vi "Get Control Information.vi"(8 "error in (no error)":errorcluster, 11 "Waveform Graph in":refnum<class "Waveform Graph.lvclass">) -> (0 "error out":errorcluster, 2 "Control Information":string[][](array[string]), 3 "Waveform Graph out":refnum<class "Waveform Graph.lvclass">)   [LabVIEW 2017, in "Localization.lvlib" / "Waveform Graph.lvclass"]
doc: "VI for override that is supposed to do go throgh the process for each control type and pull out the information that is necessary for each control.\n\nChoose Movement Consulting, LLC"
uses:
  Waveform Graph.lvclass
  C:/Apps/CMC/OpenSource/Localization/Control Info/Control Info.lvclass
  Localization.lvlib
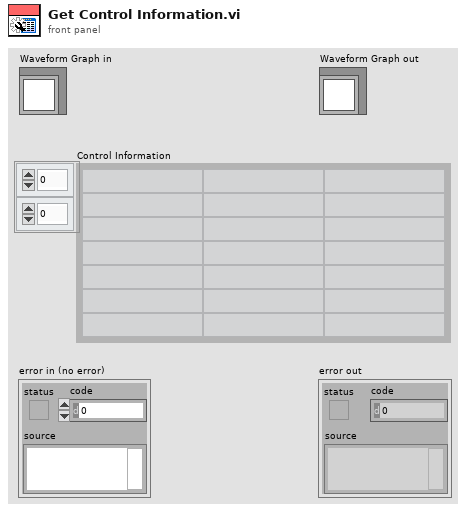
[diagram p1: front panel]
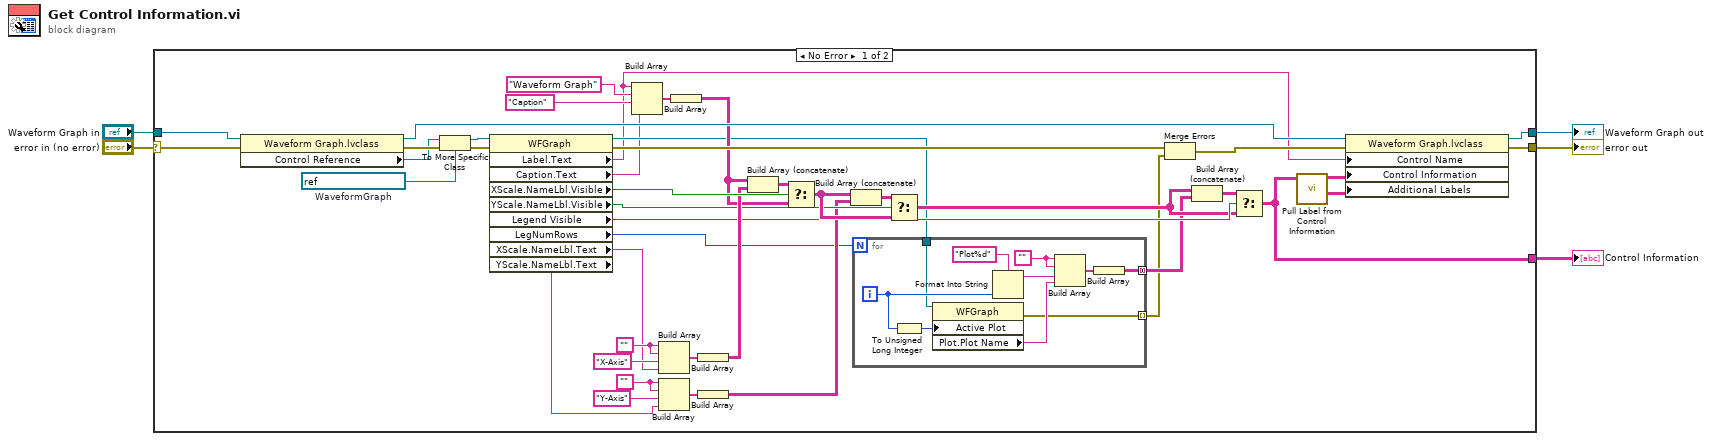
[diagram p0: block diagram]
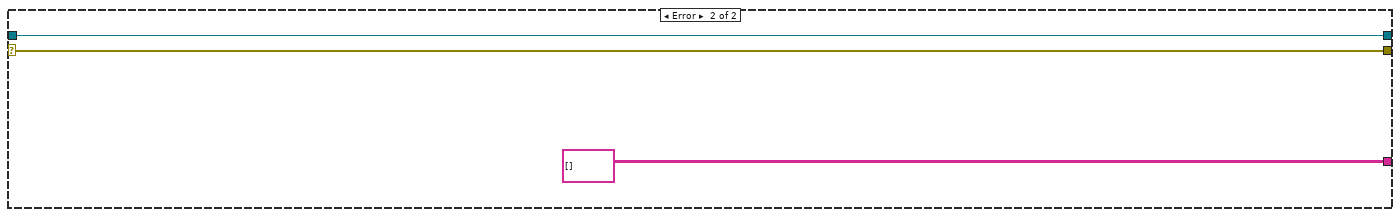
[diagram p2: hidden frame]
diagram:
  n1 = case shown="No Error" "error in (no error)" {
    selector: "error in (no error)" -> [w43 w61]
    tunnel: [w39 w61] -> w3
    tunnel: "Waveform Graph in" -> [w42 w60]
    tunnel: [w8 string[][] []] -> w2
    tunnel: [w37 w60] -> w1
    frame No Error {
      w26 = ""
      w29 = ""
      w48 = refnum<vi> refnum  # WaveformGraph
      n2 = property class="Waveform Graph.lvclass"(reference=w42, error in=w43) -> (reference out=w38:refnum<class "Waveform Graph.lvclass">, error out=w44:errorcluster, "Control Reference"=w41:refnum<vi>)
      n3 = To More Specific Class(target class=w48, reference=w41, error in=w44) -> (specific class reference=w47:refnum<vi>, error out=w45:errorcluster)
      n4 = property class="WFGraph"(reference=w47, error in=w45) -> (reference out=w13:refnum<vi>, error out=w40:errorcluster, "Label.Text"=w9:string, "Caption.Text"=w10:string, "XScale.NameLbl.Visible"=w36:bool, "YScale.NameLbl.Visible"=w22:bool, "Legend Visible"=w18:bool, "LegNumRows"=w20:u32, "XScale.NameLbl.Text"=w14:string, "YScale.NameLbl.Text"=w15:string)
      n5 = Build Array(w9, "Waveform Graph", "Caption", w10) -> (w46:string[])
      n6 = Build Array(w29, w29, "X-Axis", w14) -> (w30:string[])
      n7 = Build Array(w26, w26, "Y-Axis", w15) -> (w25:string[])
      n8 = Build Array(w46) -> (w34:string[][])
      n9 = Build Array(w30) -> (w35:string[][])
      n10 = Build Array(w25) -> (w21:string[][])
      n11 = Build Array (concatenate)(w34, w35) -> (w33:string[][])
      n12 = Select(t=w33, s=w36, f=w34) -> (s? t:f=w23:string[][])
      n13 = Build Array (concatenate)(w23, w21) -> (w24:string[][])
      n14 = for {
        N: w20 -> [_]
        tunnel: [w57] -> w16 mode=concatenating
        tunnel: w13 -> [w50]
        tunnel: [w49] -> w11 mode=indexing
        i -> [w53]
        w56 = ""
        n15 = To Unsigned Long Integer(number=w53) -> (unsigned 32bit integer=w51:u32)
        n16 = property class="WFGraph"(reference=w50, "Active Plot"=w51) -> (error out=w49:errorcluster, "Plot.Plot Name"=w52:string)  [unwired: 1 in, 1 out]
        n17 = Format Into String(format string="Plot%d", w53) -> (resulting string=w54:string)  [unwired: 2 in, 1 out]
        n18 = Build Array(w56, w56, w54, w52) -> (w58:string[])
        n19 = Build Array(w58) -> (w57:string[][])
      }
      n20 = Select(t=w24, s=w22, f=w23) -> (s? t:f=w17:string[][])
      n21 = Merge Errors(w40, w11) -> (w12:errorcluster)
      n22 = Build Array (concatenate)(w17, w16) -> (w19:string[][])
      n23 = Select(t=w19, s=w18, f=w17) -> (s? t:f=w8:string[][])
      n24 = call "Pull Label from Control Information.vi"("Control Caption Table"=w8) -> ("Additional Labels"=w6:string[][], "Control Information"=w7:string[][])  [unwired: 9 in]
      n25 = property class="Waveform Graph.lvclass"(reference=w38, error in=w12, "Control Name"=w9, "Control Information"=w7, "Additional Labels"=w6) -> (reference out=w37:refnum<class "Waveform Graph.lvclass">, error out=w39:errorcluster)
    }
    frame Error {
    }
  }
  "error out" <- w3
  "Waveform Graph out" <- w1
  "Control Information" <- w2
